vi "pathfix.vi"(4 "Current VI's Path":path) -> (1 "Fixed path":path)   [LabVIEW 2020, in "Sgraph_lib_V1.lvlib"]
doc: "André Koelewijn, feb 2020\n\nThis via will present the current VI's path\nThe effect of additional executional directories are removed.\nThe input has to be wired to the \"Current VI's path\" constant. In this way\nthe sub-vi folder setting problem is solved."
uses:
  Builds/Sgraph_lib_V1.lvlib
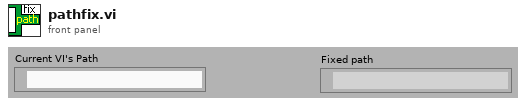
[diagram p1: front panel]
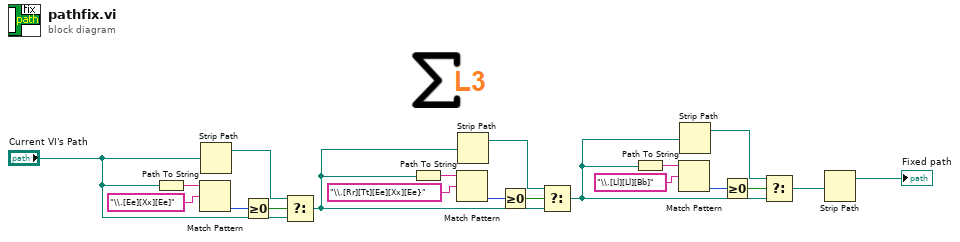
[diagram p0: block diagram]
diagram:
  n1 = Path To String(path="Current VI's Path") -> (string=w20:string)
  n2 = Match Pattern(string=w20, regular expression="\\.[Ee][Xx][Ee]") -> (offset past match=w18:i32)  [unwired: 1 in, 3 out]
  n3 = Strip Path(path="Current VI's Path") -> (stripped path=w16:path)  [unwired: 1 out]
  n4 = Greater Or Equal To 0?(x=w18) -> (x >= 0?=w17:bool)
  n5 = Select(t=w16, s=w17, f="Current VI's Path") -> (s? t:f=w10:path)
  n6 = Path To String(path=w10) -> (string=w11:string)
  n7 = Match Pattern(string=w11, regular expression="\\.[Rr][Tt][Ee][Xx][Ee}") -> (offset past match=w13:i32)  [unwired: 1 in, 3 out]
  n8 = Strip Path(path=w10) -> (stripped path=w15:path)  [unwired: 1 out]
  n9 = Greater Or Equal To 0?(x=w13) -> (x >= 0?=w14:bool)
  n10 = Select(t=w15, s=w14, f=w10) -> (s? t:f=w4:path)
  n11 = Path To String(path=w4) -> (string=w5:string)
  n12 = Match Pattern(string=w5, regular expression="\\.[Ll][Ll][Bb]") -> (offset past match=w7:i32)  [unwired: 1 in, 3 out]
  n13 = Strip Path(path=w4) -> (stripped path=w9:path)  [unwired: 1 out]
  n14 = Greater Or Equal To 0?(x=w7) -> (x >= 0?=w8:bool)
  n15 = Select(t=w9, s=w8, f=w4) -> (s? t:f=w3:path)
  n16 = Strip Path(path=w3) -> (stripped path=→"Fixed path":path)  [unwired: 1 out]
